vi "Connect to Data Server.vi"(8 "error in (no error)":errorcluster, 9 "timeout ms (60000)":i32=60000, 11 "server address":string) -> (0 "error out":errorcluster, 1 "timed out?":bool, 2 "Framework Configuration":refnum<class "Framework Configuration.lvclass">, 3 "server ID":refnum<k5>)   [LabVIEW 2019, in "DSF Core.lvlib"]
uses:
  DSF Core.lvlib
  Configuration/Core/Framework/Framework Configuration.lvclass
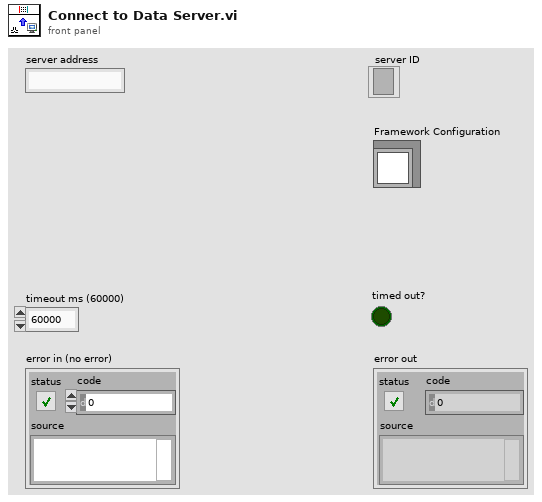
[diagram p1: front panel]
types:
  T1 = enum16{"big-endian, network order", "native, host order", "little-endian"}
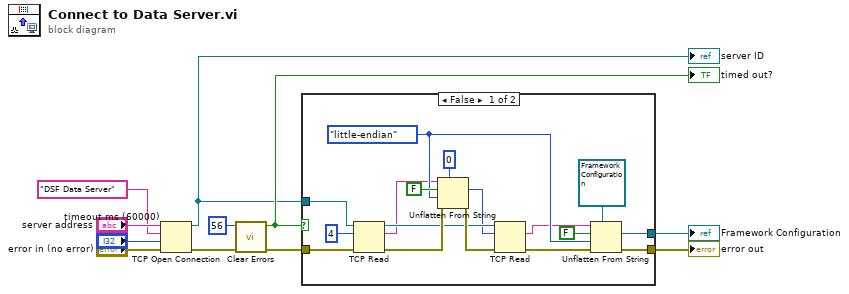
[diagram p0: block diagram]
diagram:
  n1 = TCP Open Connection(address="server address", remote port or service name="DSF Data Server" ("address"), timeout ms (60000)="timeout ms (60000)", error in (no error)="error in (no error)") -> (connection ID=w2:refnum<k5>, error out=w6:errorcluster)  [unwired: 1 in]
  "server ID" <- w2
  n2 = call <vilib>:"Clear Errors.vi"("error in (no error)"=w6, "specific error code to clear (0: all)"=56) -> ("error out"=w5:errorcluster, "specific error cleared?"=w4:bool)  [unwired: 4 in]
  "timed out?" <- w4
  n3 = case shown="False" w4 {
    tunnel: w5 -> [w28 w29]
    tunnel: [w18 w29] -> w3
    tunnel: w2 -> [w27 _]
    tunnel: [w16 _] -> w1
    frame False {
      w17 = T1."little-endian" ("byte order (0:big-endian, network order)")
      n4 = TCP Read(connection ID=w27, bytes to read=4, error in (no error)=w28) -> (connection ID out=w21:refnum<k5>, data out=w15:string, error out=w25:errorcluster)  [unwired: 2 in]
      n5 = Unflatten From String(type=0, binary string=w15, data includes array or string size? (T)=FALSE, byte order (0:big-endian, network order)=w17, error in (no error)=w25) -> (value=w13:i32, error out=w22:errorcluster)  [unwired: 1 out]
      n6 = TCP Read(connection ID=w21, bytes to read=w13, error in (no error)=w22) -> (data out=w14:string, error out=w19:errorcluster)  [unwired: 2 in, 1 out]
      n7 = Unflatten From String(type=refnum<class "Framework Configuration.lvclass"> refnum ("DSF Core.lvlib:Framework Configuration.lvclass"), binary string=w14, data includes array or string size? (T)=FALSE, byte order (0:big-endian, network order)=w17, error in (no error)=w19) -> (value=w16:refnum<class "Framework Configuration.lvclass">, error out=w18:errorcluster)  [unwired: 1 out]
    }
    frame True {
    }
  }
  "error out" <- w3
  "Framework Configuration" <- w1
